vi "Main.vi"() -> ()   [LabVIEW 2019, in "Model.lvlib"]
doc: "This template is based off of the Queued Message Handler design pattern and the Queued Message Handler project template that ships with LabVIEW.\n\nThe main difference is that the queue is private to this module and communication between modules is performed via Broadcast and Request events.\n\nRequest events are wrapped in public API methods and are handled in the Event Handling Loop (EHL) of this VI. Any module can register for Broadcast events sent by this module. The EHL generates messages based on user interface actions.\n\nThe Message Handling Loop (MHL) processes messages generated by the EHL, or by other messages. The messages are string values, so new messages can be added easily to the Message Cases case structure in the MHL. Each message cluster can also provide an optional value for Message Data, which is a variant that can be converted to whatever message-specific data is required.\n_____\nBased on Delacor QMH Project Template 4.2.1.64."
uses:
  Model.lvlib
  <vilib>/Delacor/Delacor QMH/Libraries/Module Admin_class/Delacor_lib_QMH_Module Admin.lvclass
  Module Data--cluster.ctl
  <vilib>/Delacor/Delacor QMH/Libraries/Message Queue_class/Delacor_lib_QMH_Message Queue.lvclass/Delacor_lib_QMH_Message Queue.ctl
  Stop Argument--cluster.ctl
  <vilib>/Delacor/Delacor QMH/Libraries/Module Admin_class/Delacor_lib_QMH_Module Admin.lvclass/Delacor_lib_QMH_Module Admin.ctl
  <vilib>/Delacor/Delacor QMH/Libraries/Message Queue_class/Delacor_lib_QMH_Enqueue Message (Single).vi
  <vilib>/Delacor/Delacor QMH/Libraries/Module Admin_class/Delacor_lib_QMH_Get External Launch.vi
  <vilib>/Utility/error.llb/Error Cluster From Error Code.vi
  <vilib>/ErrorRing/Error Ring.xnode
  <vilib>/Delacor/Delacor QMH/Libraries/Message Queue_class/Delacor_lib_QMH_Message Queue.lvclass
  Stock/Stock.lvlib
  Display/Display.lvlib
  Keypad/Keypad.lvlib
  Money/Money.lvlib
panel:
  in  "Power":bool
  in  "Simulate MHL Error":bool
  in  "Simulate EHL Error":bool
  in  "Module Admin":refnum<class "Delacor_lib_QMH_Module Admin.lvclass">
  out "Status":string
  out "error out":errorcluster
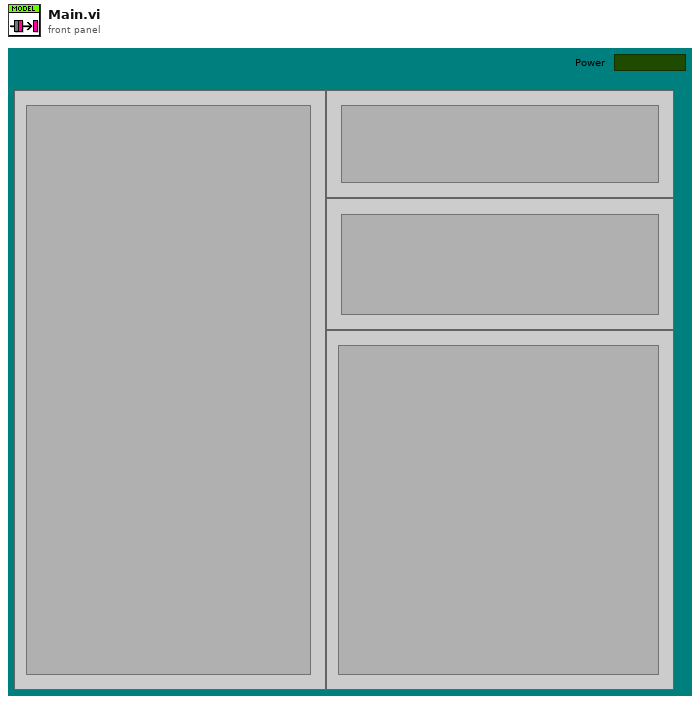
[diagram p1: front panel]
types:
  T1 = typedef "Model.lvlib/Request Events--cluster.ctl" = cluster{"Stop Module":refnum<user-event>, "Show Panel":refnum<user-event>, "Hide Panel":refnum<user-event>, "Get Module Execution Status":refnum<user-event>, "Show Diagram":refnum<user-event>}
  T2 = typedef "Stock.lvlib/Broadcast Events--cluster.ctl" = cluster{"Module Did Init":refnum<user-event>, "Status Updated":refnum<user-event>, "Error Reported":refnum<user-event>, "Module Did Stop":refnum<user-event>, "Update Module Execution Status":refnum<user-event>}
  T3 = typedef "Display.lvlib/Broadcast Events--cluster.ctl" = cluster{"Module Did Init":refnum<user-event>, "Status Updated":refnum<user-event>, "Error Reported":refnum<user-event>, "Module Did Stop":refnum<user-event>, "Update Module Execution Status":refnum<user-event>}
  T4 = typedef "Keypad.lvlib/Broadcast Events--cluster.ctl" = cluster{"Module Did Init":refnum<user-event>, "Status Updated":refnum<user-event>, "Error Reported":refnum<user-event>, "Module Did Stop":refnum<user-event>, "Update Module Execution Status":refnum<user-event>, "Product Selected":refnum<user-event>, "Cancel Request":refnum<user-event>}
  T5 = typedef "Money.lvlib/Broadcast Events--cluster.ctl" = cluster{"Module Did Init":refnum<user-event>, "Status Updated":refnum<user-event>, "Error Reported":refnum<user-event>, "Module Did Stop":refnum<user-event>, "Update Module Execution Status":refnum<user-event>, "Money Entered":refnum<user-event>, "Money Refunded":refnum<user-event>}
  T6 = typedef "Model.lvlib/Module Data--cluster.ctl" = cluster{"Status":string}
  T7 = enum32{"invalid lock state", "Not Locked", "Locked (No Password)", "Password-protected"}
  T8 = typedef "Model.lvlib/Stop Argument--cluster.ctl" = cluster{"Origin":string, "Exit via Stop Module Req?":bool, "Wait for Module to stop?":bool}
  T9 = enum32{"Invalid", "Standard", "Closed", "Hidden", "Minimized", "Maximized"}
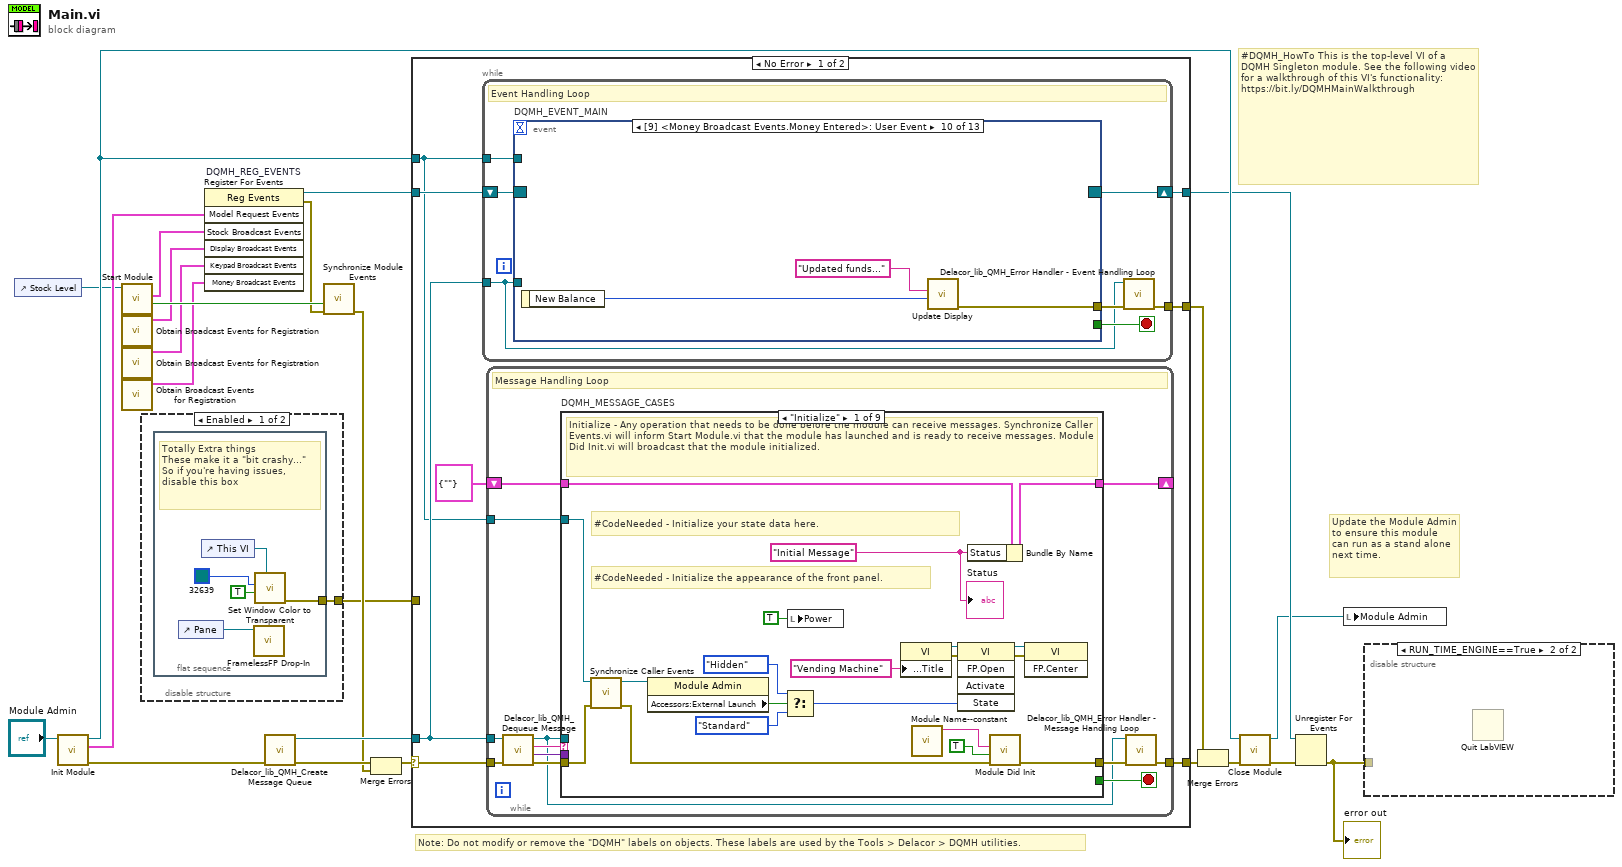
[diagram p0: block diagram]
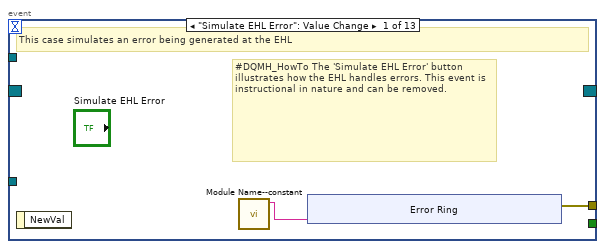
[diagram p4: hidden frame]
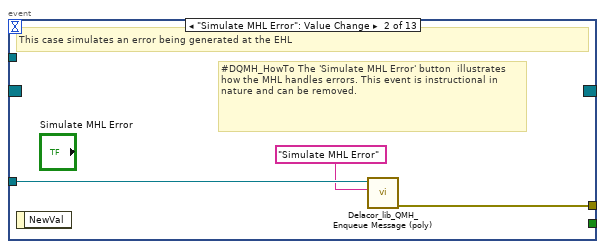
[diagram p5: hidden frame]
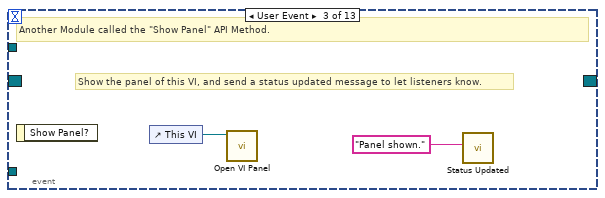
[diagram p6: hidden frame]
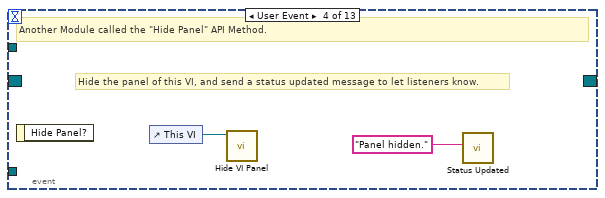
[diagram p7: hidden frame]
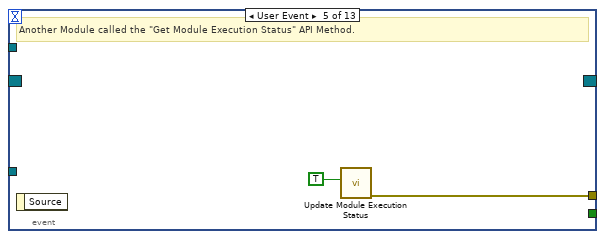
[diagram p8: hidden frame]
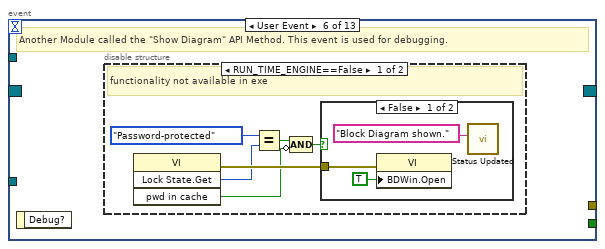
[diagram p9: hidden frame]
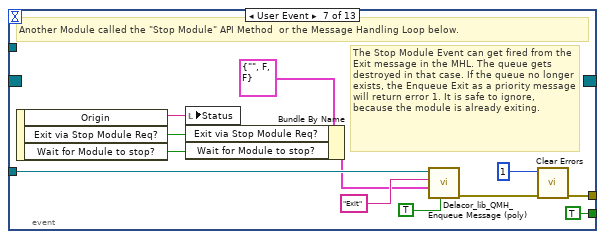
[diagram p12: hidden frame]
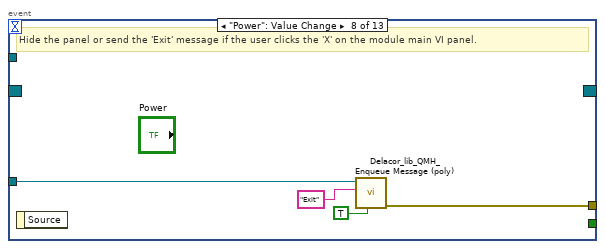
[diagram p13: hidden frame]
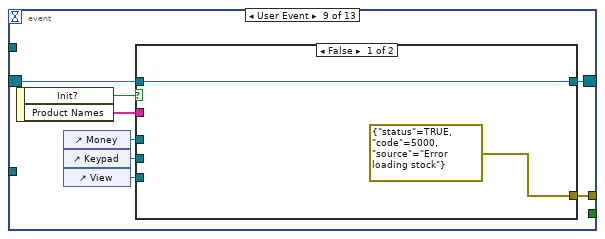
[diagram p14: hidden frame]
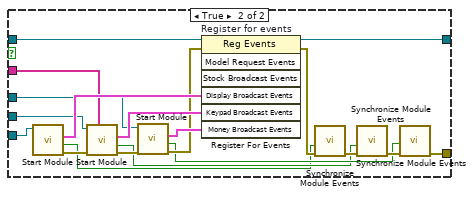
[diagram p15: hidden frame]
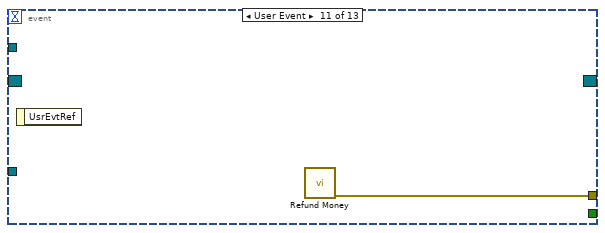
[diagram p16: hidden frame]
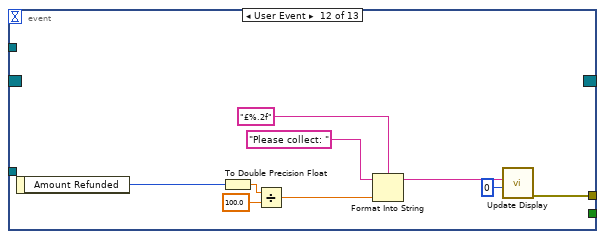
[diagram p17: hidden frame]
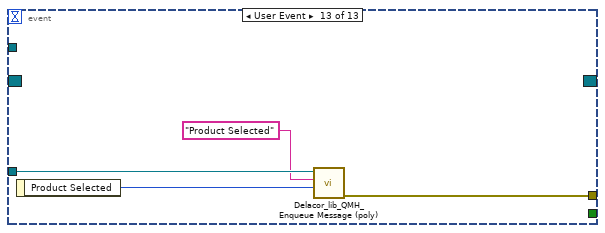
[diagram p18: hidden frame]
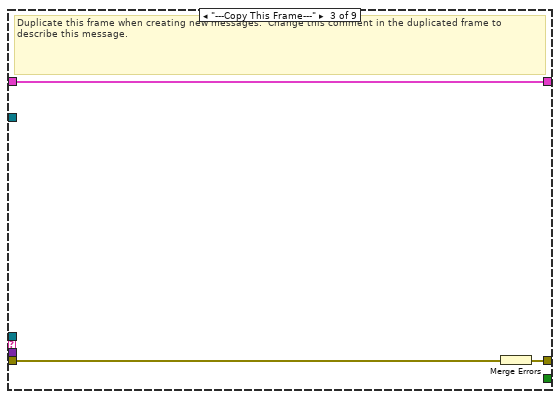
[diagram p20: hidden frame]
diagram:
  # "#DQMH_HowTo This is the top-level VI of a DQMH Singleton module. See the following video for a walkthrough of this VI's functionality: https://bit.ly/DQMHMainWalkthrough"
  # "Note: Do not modify or remove the \"DQMH\" labels on objects. These labels are used by the Tools > Delacor > DQMH utilities."
  # "Update the Module Admin to ensure this module can run as a stand alone next time."
  n1 = control-ref of="Stock Level"() -> (w3:refnum<vi>)
  n2 = call "Init Module.vi"("Singleton Module Admin in"="Module Admin") -> ("error out"=w23:errorcluster, "Model Request Events"=w14:T1, "Singleton Module Admin out"=w17:refnum<class "Delacor_lib_QMH_Module Admin.lvclass">)  [unwired: 8 in]
  n3 = call "Start Module.vi"("Subpanel Ref"=w3) -> ("Wait for Event Sync?"=w9:bool, "Stock Broadcast Events"=w10:T2)  [unwired: 7 in, 2 out]
  n4 = call "Obtain Broadcast Events for Registration.vi"() -> ("Display Broadcast Events"=w6:T3)  [unwired: 9 in, 2 out]
  n5 = call "Obtain Broadcast Events for Registration.vi"() -> ("Keypad Broadcast Events"=w5:T4)  [unwired: 9 in, 2 out]
  n6 = call "Obtain Broadcast Events for Registration.vi"() -> ("Money Broadcast Events"=w4:T5)  [unwired: 9 in, 2 out]
  n7 = disable-structure shown="Enabled" {
    disable-tunnel: [w25 _] -> w1
    frame Enabled {
      n8 = flat-sequence {
        tunnel: [w26] -> w25
        frame #0 {
          # "Totally Extra things\nThese make it a \"bit crashy...\"\nSo if you're having issues, disable this box"
          n9 = control-ref of="Pane"() -> (w30:refnum<vi>)
          n10 = control-ref of="This VI"() -> (w29:refnum<vi>)
          n11 = call "FramelessFP Drop-In.vi"("Pane in"=w30) -> ()  [unwired: 10 in, 1 out]
          n12 = call "Set Window Color to Transparent.vi"("Calling VI's reference"=w29, "Activate"=TRUE, "Color to Replace"=u32 32639) -> ("error out"=w26:errorcluster)  [unwired: 5 in]
        }
      }
    }
    frame Disabled {
    }
  }
  n13 = register-events "DQMH_REG_EVENTS"(w14, w10, w6, w5, w4) -> (reference out=w15:refnum<event-registration>, error out=w8:errorcluster)  [unwired: 2 in]
  n14 = call <vilib>:"Delacor_lib_QMH_Create Message Queue.vi"("error in (no error)"=w23) -> ("error out"=w19:errorcluster, "Message Queue"=w13:refnum<class "Delacor_lib_QMH_Message Queue.lvclass">)  [unwired: 9 in]
  n15 = call "Synchronize Module Events.vi"("error in (no error)"=w8, "Wait for Event Sync?"=w9) -> ("error out"=w7:errorcluster)  [unwired: 9 in]
  n16 = Merge Errors(w19, w7) -> (w18:errorcluster)
  n17 = case shown="No Error" w18 {
    selector: w18 -> [w36 w241]
    tunnel: [w38 w241] -> w24
    tunnel: [w35 w238] -> w16
    tunnel: w15 -> [w33 w238]
    tunnel: w13 -> [w32 _]
    tunnel: [w37 _] -> w21
    tunnel: w17 -> [w31 w234]
    tunnel: w1 -> [_ _]
    frame No Error {
      n18 = while {
        tunnel: w32 -> [w39]
        shift-right: [w42] -> w35
        shift-left: w33 -> [w43]
        tunnel: [w44] -> w37
        tunnel: w31 -> [w40]
        stop <- w41 stop-if-true
        # "Event Handling Loop"
        n19 = event "DQMH_EVENT_MAIN" shown="[9] <Money Broadcast Events.Money Entered>: User Event" {
          selector: w43 -> [_ _ _ _ _ _ _ _ w93 _ _ _ _]
          dyn-events: [_ _ _ _ _ _ _ _ w92 _ _ _ _] -> w42
          timeout: _ -> [_ _ _ _ _ _ _ _ _ _ _ _ _]
          tunnel: [_ _ _ _ _ _ TRUE ("Discard?") _ _ _ _ _ _] -> w41
          tunnel: w39 -> [_ w56 _ _ _ _ w80 w87 _ _ _ _ w134]
          tunnel: [w47 w57 _ _ w63 _ w83 w88 w95 w120 w121 w130 w133] -> w45
          tunnel: w40 -> [_ _ _ _ _ _ _ _ _ _ _ _ _]
          event "Simulate EHL Error": Value Change {
            # "#DQMH_HowTo The 'Simulate EHL Error' button  illustrates how the EHL handles errors. This event is instructional in nature and can be removed."
            # "This case simulates an error being generated at the EHL"
            n20 = event-data() -> ()  [unwired: 1 in, 1 out]
            n21 = call "Module Name--constant.vi"() -> ("Module Name"=w46:string)  [unwired: 11 in]
            n22 = xnode "Error Ring"("parameter 0"=w46) -> ("error out"=w47:errorcluster)
          }
          event "Simulate MHL Error": Value Change {
            # "#DQMH_HowTo The 'Simulate MHL Error' button  illustrates how the MHL handles errors. This event is instructional in nature and can be removed."
            # "This case simulates an error being generated at the EHL"
            n23 = event-data() -> ()  [unwired: 1 in, 1 out]
            n24 = call-poly <vilib>:"Delacor_lib_QMH_Enqueue Message (poly).vi"("Message"="Simulate MHL Error", "Message Queue in"=w56) -> ("error out"=w57:errorcluster)  [unwired: 8 in, 1 out]
          }
          event User Event {
            # "Show the panel of this VI, and send a status updated message to let listeners know."
            # "Another Module called the \"Show Panel\" API Method."
            n25 = event-data() -> ()  [unwired: 1 in, 1 out]
            n26 = control-ref of="This VI"() -> (w59:refnum<vi>)
            n27 = call "Open VI Panel.vi"("VI"=w59) -> ()  [unwired: 10 in, 1 out]
            n28 = call "Status Updated.vi"("Status"="Panel shown." ("format string")) -> ()  [unwired: 10 in, 1 out]
          }
          event User Event {
            # "Hide the panel of this VI, and send a status updated message to let listeners know."
            # "Another Module called the \"Hide Panel\" API Method."
            n29 = event-data() -> ()  [unwired: 1 in, 1 out]
            n30 = control-ref of="This VI"() -> (w61:refnum<vi>)
            n31 = call "Hide VI Panel.vi"("VI"=w61) -> ()  [unwired: 10 in, 1 out]
            n32 = call "Status Updated.vi"("Status"="Panel hidden." ("format string")) -> ()  [unwired: 10 in, 1 out]
          }
          event User Event {
            # "Another Module called the \"Get Module Execution Status\" API Method."
            n33 = event-data() -> ()  [unwired: 1 in, 1 out]
            n34 = call "Update Module Execution Status.vi"("Running?"=TRUE) -> ("error out"=w63:errorcluster)  [unwired: 10 in]
          }
          event User Event {
            # "Another Module called the \"Show Diagram\" API Method. This event is used for debugging."
            n35 = event-data() -> ()  [unwired: 1 in, 1 out]
            n36 = disable-structure shown="RUN_TIME_ENGINE==False" {
              frame condition #0 (active) {
                # "functionality not available in exe"
                n37 = invoke class="VI" method="Lock State.Get"() -> (error out=w69:errorcluster, "Get Lock State"=w68:T7, "pwd in cache"=w65:bool)  [unwired: 4 in, 1 out]
                n38 = Equal?(x=T7."Password-protected", y=w68) -> (x = y?=w66:bool)
                n39 = Compound Arithmetic op=AND(w66, invert w65) -> (w64:bool)
                n40 = case shown="False" w64 {
                  tunnel: w69 -> [w72 _]
                  frame False {
                    n41 = property class="VI"(error in=w72, "BDWin.Open"=TRUE ("Block Diagram Window:Open")) -> ()  [unwired: 1 in, 2 out]
                    n42 = call "Status Updated.vi"("Status"="Block Diagram shown." ("format string")) -> ()  [unwired: 10 in, 1 out]
                  }
                  frame True {
                    # "Password-protected VI, and the password is not in the cache. Do not show the diagram."
                  }
                }
              }
              frame condition #1 {
              }
            }
          }
          event User Event {
            # "The Stop Module Event can get fired from the Exit message in the MHL. The queue gets destroyed in that case. If the queue no longer exists, the Enqueue Exit as a priority message will return error 1. It is safe to ignore, because the module is already exiting."
            # "Another Module called the \"Stop Module\" API Method  or the Message Handling Loop below."
            n43 = event-data() -> ("Origin"=w79:string, "Exit via Stop Module Req?"=w75:bool, "Wait for Module to stop?"=w74:bool)  [unwired: 1 in]
            n44 = local write "Status"(w79) -> ()
            n45 = Bundle By Name(cluster=T8 {"Origin"="", "Exit via Stop Module Req?"=FALSE, "Wait for Module to stop?"=FALSE} ("Stop Argument"), "Exit via Stop Module Req?"=w75, "Wait for Module to stop?"=w74) -> (w73:T8)
            n46 = call-poly <vilib>:"Delacor_lib_QMH_Enqueue Message (poly).vi"("Priority Message? (F)"=TRUE, "Message Data"=w73, "Message"="Exit", "Message Queue in"=w80) -> ("error out"=w84:errorcluster)  [unwired: 6 in, 1 out]
            n47 = call <vilib>:"Clear Errors.vi"("error in (no error)"=w84, "specific error code to clear (0: all)"=1) -> ("error out"=w83:errorcluster)  [unwired: 4 in, 1 out]
          }
          event "Power": Value Change {
            # "Hide the panel or send the 'Exit' message if the user clicks the 'X' on the module main VI panel."
            n48 = event-data() -> ()  [unwired: 1 in, 1 out]
            n49 = call-poly <vilib>:"Delacor_lib_QMH_Enqueue Message (poly).vi"("Priority Message? (F)"=TRUE, "Message"="Exit", "Message Queue in"=w87) -> ("error out"=w88:errorcluster)  [unwired: 7 in, 1 out]
          }
          event User Event {
            n50 = event-data() -> ("Init?"=w96:bool, "Product Names"=w94:string[])  [unwired: 1 in]
            n51 = control-ref of="Money"() -> (w91:refnum<vi>)
            n52 = control-ref of="Keypad"() -> (w90:refnum<vi>)
            n53 = control-ref of="View"() -> (w89:refnum<vi>)
            n54 = case shown="False" w96 {
              tunnel: [errorcluster {"status"=TRUE, "code"=5000, "source"="Error loading stock"} ("error constant") w106] -> w95
              tunnel: w94 -> [_ w102]
              tunnel: w93 -> [w97 w117]
              tunnel: [w97 w116] -> w92
              tunnel: w91 -> [_ w99]
              tunnel: w90 -> [_ w100]
              tunnel: w89 -> [_ w101]
              frame False {
              }
              frame True {
                n55 = call "Start Module.vi"("Subpanel Ref"=w101) -> ("error out"=w112:errorcluster, "Wait for Event Sync?"=w103:bool, "Display Broadcast Events"=w115:T3)  [unwired: 7 in, 1 out]
                n56 = call "Start Module.vi"("Product Names"=w102, "error in (no error)"=w112, "Subpanel Ref"=w100) -> ("error out"=w111:errorcluster, "Wait for Event Sync?"=w104:bool, "Keypad Broadcast Events"=w114:T4)  [unwired: 5 in, 1 out]
                n57 = call "Start Module.vi"("error in (no error)"=w111, "Subpanel Ref"=w99) -> ("error out"=w110:errorcluster, "Wait for Event Sync?"=w105:bool, "Money Broadcast Events"=w113:T5)  [unwired: 6 in, 1 out]
                n58 = register-events "Register for events"(reference=w117, error in=w110, w115, w114, w113) -> (reference out=w116:refnum<event-registration>, error out=w109:errorcluster)  [unwired: 2 in]
                n59 = call "Synchronize Module Events.vi"("error in (no error)"=w109, "Wait for Event Sync?"=w103) -> ("error out"=w108:errorcluster)  [unwired: 9 in]
                n60 = call "Synchronize Module Events.vi"("error in (no error)"=w108, "Wait for Event Sync?"=w104) -> ("error out"=w107:errorcluster)  [unwired: 9 in]
                n61 = call "Synchronize Module Events.vi"("error in (no error)"=w107, "Wait for Event Sync?"=w105) -> ("error out"=w106:errorcluster)  [unwired: 9 in]
              }
            }
          }
          event User Event {
            n62 = event-data() -> ("New Balance"=w119:u32)  [unwired: 1 in]
            n63 = call "Update Display.vi"("Balance"=w119, "Message to display"="Updated funds...") -> ("error out"=w120:errorcluster)  [unwired: 9 in]
          }
          event User Event {
            n64 = event-data() -> ()  [unwired: 1 in, 1 out]
            n65 = call "Refund Money.vi"() -> ("error out"=w121:errorcluster)  [unwired: 11 in]
          }
          event User Event {
            n66 = event-data() -> ("Amount Refunded"=w124:u32)  [unwired: 1 in]
            n67 = To Double Precision Float(number=w124) -> (double precision float=w127:dbl)
            n68 = Divide(x=w127, y=100.0) -> (x/y=w125:dbl)
            n69 = Format Into String(format string="£%.2f", initial string="Please collect: ", w125) -> (resulting string=w123:string)  [unwired: 1 in, 1 out]
            n70 = call "Update Display.vi"("Balance"=u32 0, "Message to display"=w123) -> ("error out"=w130:errorcluster)  [unwired: 9 in]
          }
          event User Event {
            n71 = event-data() -> ("Product Selected"=w131:u32)  [unwired: 1 in]
            n72 = call-poly <vilib>:"Delacor_lib_QMH_Enqueue Message (poly).vi"("Message Data"=w131, "Message"="Product Selected", "Message Queue in"=w134) -> ("error out"=w133:errorcluster)  [unwired: 7 in, 1 out]
          }
        }
        n73 = call-dynamic "Delacor_lib_QMH_Error Handler - Event Handling Loop.vi"("error in (no error)"=w45, "Message Queue in"=w39) -> ("dup error in"=w44:errorcluster)  [unwired: 8 in, 1 out]
      }
      n74 = while {
        tunnel: w32 -> [w137]
        shift-right: [w141] -> _
        shift-left: T6 {"Status"=""} ("Data Cluster") -> [w142]
        tunnel: w36 -> [w145]
        tunnel: [w143] -> w38
        tunnel: w31 -> [w135]
        stop <- w140 stop-if-true
        # "Message Handling Loop"
        n75 = call-dynamic "Delacor_lib_QMH_Dequeue Message.vi"("error in (no error)"=w145, "Message Queue in"=w137) -> ("error out"=w144:errorcluster, "Message Data"=w138:variant, "Message"=w139:string, "Message Queue out"=w136:refnum<class "Delacor_lib_QMH_Message Queue.lvclass">)  [unwired: 6 in]
        n76 = case "DQMH_MESSAGE_CASES" shown="\"Initialize\"" w139 {
          selector: w139 -> [_ _ _ _ _ _ _ _ w221]
          tunnel: w136 -> [_ _ _ _ _ _ w196 w213 _]
          tunnel: w144 -> [w164 w168 w171 w176 w180 w185 w203 w219 w223]
          tunnel: [w162 w168 w170 w172 w180 w184 w199 w216 w224] -> w146
          tunnel: w142 -> [w154 w167 w169 w178 w179 w182 w198 w212 w222]
          tunnel: [w153 w167 w169 w178 w179 w182 w198 w212 w222] -> w141
          tunnel: [_ _ _ _ _ _ _ w211 _] -> w140
          tunnel: w138 -> [_ _ _ w177 _ _ w197 w210 _]
          tunnel: w135 -> [w155 _ _ _ _ _ w195 w205 _]
          frame "Initialize" {
            w149 = "Initial Message" ("Initial Message")
            # "#CodeNeeded - Initialize the appearance of the front panel."
            # "#CodeNeeded - Initialize your state data here."
            # "Initialize - Any operation that needs to be done before the module can receive messages. Synchronize Caller Events.vi will inform Start Module.vi that the module has launched and is ready to receive messages. Module Did Init.vi will broadcast that the module initialized."
            n77 = call "Synchronize Caller Events.vi"("error in (no error)"=w164, "Singleton Module Admin in"=w155) -> ("error out"=w163:errorcluster, "Singleton Module Admin out"=w150:refnum<class "Delacor_lib_QMH_Module Admin.lvclass">)  [unwired: 8 in]
            n78 = property class="Module Admin"(reference=w150) -> ("Accessors:External Launch"=w159:bool)  [unwired: 1 in, 2 out]
            n79 = Select(t=T9."Hidden" ("State"), s=w159, f=T9."Standard" ("State")) -> (s? t:f=w156:T9)
            n80 = local write "Power"(TRUE ("Power")) -> ()
            n81 = property class="VI"("Front Panel.Title"="Vending Machine" ("Front Panel Window:Title")) -> (reference out=w161:refnum<vi>, error out=w166:errorcluster)  [unwired: 2 in]
            n82 = call "Module Name--constant.vi"() -> ("Module Name"=w151:string)  [unwired: 11 in]
            n83 = invoke class="VI" method="FP.Open"(reference=w161, error in=w166, "State"=w156) -> (reference out=w160:refnum<vi>, error out=w165:errorcluster)  [unwired: 2 in, 3 out]
            n84 = Bundle By Name(cluster=w154, "Status"=w149) -> (w153:T6)
            n85 = call "Module Did Init.vi"("error in (no error)"=w163, "Initialized?"=TRUE, "Origin"=w151) -> ("error out"=w162:errorcluster)  [unwired: 8 in]
            n86 = invoke class="VI" method="FP.Center"(reference=w160, error in=w165) -> ()  [unwired: 1 in, 3 out]
            "Status" <- w149
          }
          frame "--- Module Specific ---" {
            # "Separator -- The following cases handle messages specific to this Module."
          }
          frame "---Copy This Frame---" {
            # "Duplicate this frame when creating new messages.  Change this comment in the duplicated frame to describe this message."
            n87 = Merge Errors(w171) -> (w170:errorcluster)
          }
          frame "Product Selected" {
            # "All in one VI to reduce the risk of race conditions"
            # "Check Stock Level, Check Balance\nOutputs: Not in stock,  Insufficient Funds, Accepted (Reduce Stock and Balance"
            n88 = Variant To Data(error in=w176, type=u32 0 ("Product Selected"), Variant=w177) -> (data=w174:u32, error out=w173:errorcluster)
            n89 = call "Despence Product.vi"("error in (no error)"=w173, "Stock Item"=w174) -> ("error out"=w172:errorcluster)  [unwired: 9 in]
          }
          frame "--- Exit and Error Handling---" {
            # "Separator - The following cases handle errors and exit messages."
          }
          frame "Simulate MHL Error" {
            # "#DQMH_HowTo The 'Simulate MHL Error' button  illustrates how the MHL handles errors. This event is instructional in nature and can be removed."
            # "Simulate an error occurring at the MHL"
            n90 = call "Module Name--constant.vi"() -> ("Module Name"=w181:string)  [unwired: 11 in]
            n91 = xnode "Error Ring"("parameter 0"=w181) -> ("error out"=w183:errorcluster)
            n92 = Merge Errors(w185, w183) -> (w184:errorcluster)
          }
          frame "Error" {
            # "If the module is running standalone, then pop up an error dialog and call the \"Exit\" message."
            # "#CodeRecommended - If you ever change the name of this \"Error\" message, you'll need to update the name in the Check Loop Error.vi as well."
            # "#CodeRecommended - If the module is running in standalone mode (External Launch = FALSE), this code will pop up an error dialog and call the 'Exit' message if an error occurs. Add more fine-grained error handling here."
            # "Error - Check the error message data and respond accordingly. This message is sent by the \"Error Handler\" VIs at the end of each loop in this application."
            n93 = property class="Module Admin" props=["Accessors:External Launch"](reference=w195) -> ()  [unwired: 1 in, 3 out]
            n94 = Variant To Data(error in=w203, type=errorcluster {"status"=FALSE, "code"=0, "source"=""} ("error constant"), Variant=w197) -> (data=w204:errorcluster, error out=w201:errorcluster)
            n95 = call "Error Reported.vi"("Error"=w204) -> ()  [unwired: 10 in, 1 out]
            n96 = call <vilib>:"Simple Error Handler.vi"("error in (no error)"=w204) -> ()  [unwired: 4 in, 5 out]
            n97 = call-poly <vilib>:"Delacor_lib_QMH_Enqueue Message (poly).vi"("Priority Message? (F)"=TRUE, "Message"="Exit", "Message Queue in"=w196) -> ("error out"=w200:errorcluster)  [unwired: 7 in, 1 out]
            n98 = Merge Errors(w201, w200) -> (w199:errorcluster)
            n99 = local write "error out"(w199) -> ()
          }
          frame "Exit" {
            w209 = 91  # 91: not all Exit messages will have an argument
            w211 = TRUE  # Stop the VI
            # "Release the message queue reference"
            # "Exit - Exit the application."
            n100 = Variant To Data(error in=w219, type=T8 {"Origin"="", "Exit via Stop Module Req?"=FALSE, "Wait for Module to stop?"=FALSE} ("Stop Argument"), Variant=w210) -> (data=w207:T8, error out=w215:errorcluster)
            n101 = call <vilib>:"Clear Errors.vi"("error in (no error)"=w215, "specific error code to clear (0: all)"=w209) -> ("error out"=w218:errorcluster)  [unwired: 4 in, 1 out]
            n102 = control-ref of="This VI"() -> (w206:refnum<vi>)
            n103 = call-dynamic "Delacor_lib_QMH_Release Message Queue.vi"("error in (no error)"=w218, "Message Queue"=w213) -> ("error out"=w217:errorcluster)  [unwired: 9 in]
            n104 = call "Handle Exit.vi"("Stop Argument"=w207, "Admin in"=w205, "VI reference"=w206) -> ("error out"=w214:errorcluster)  [unwired: 7 in, 1 out]
            n105 = Merge Errors(w217, w214) -> (w216:errorcluster)
            n106 = call "Stop Module.vi"() -> ()  [unwired: 11 in, 1 out]
            n107 = call "Stop Module.vi"() -> ()  [unwired: 11 in, 1 out]
            n108 = call "Stop Module.vi"() -> ()  [unwired: 11 in, 1 out]
            n109 = call "Stop Module.vi"() -> ()  [unwired: 11 in, 1 out]
          }
          frame Default {
            # "'Default' case only runs if there is a message that isn't defined in any of the other cases.  Output a programming error."
            n110 = call "Module Name--constant.vi"() -> ("Module Name"=w220:string)  [unwired: 11 in]
            n111 = xnode "Error Ring"("parameter 0"=w221, "parameter 1"=w220) -> ("error out"=w225:errorcluster)
            n112 = Merge Errors(w223, w225) -> (w224:errorcluster)
          }
        }
        n113 = call-dynamic "Delacor_lib_QMH_Error Handler - Message Handling Loop.vi"("error in (no error)"=w146, "Message Queue in"=w136) -> ("dup error in"=w143:errorcluster)  [unwired: 8 in, 1 out]
      }
    }
    frame Error {
      # "Synchronize Caller Events.vi will inform Start Module.vi that the module has launched and will let the code calling Start Module.vi register for broadcasts and would permit the caller receive the broadcast that an error occurred at launch time."
      n114 = call "Synchronize Caller Events.vi"("Singleton Module Admin in"=w234) -> ("error out"=w239:errorcluster)  [unwired: 9 in, 1 out]
      n115 = call "Module Name--constant.vi"() -> ("Module Name"=w237:string)  [unwired: 11 in]
      n116 = Format Into String(format string="An error occurred during initialization. %s is no longer running.", w237) -> (resulting string=w235:string)  [unwired: 2 in, 1 out]
      n117 = Merge Errors(w241, w239) -> (w240:errorcluster)
      n118 = call "Error Reported.vi"("Additional Information"=w235, "Error"=w240) -> ()  [unwired: 9 in, 1 out]
    }
  }
  n119 = Merge Errors(w21, w24) -> (w20:errorcluster)
  n120 = call "Close Module.vi"("error in (no error)"=w20, "Module Admin in"=w17) -> ("error out"=w22:errorcluster, "Module Admin out"=w11:refnum<class "Delacor_lib_QMH_Module Admin.lvclass">)  [unwired: 7 in, 1 out]
  n121 = Unregister For Events(event registration refnum=w16, error in=w22) -> (error out=w2:errorcluster)
  "error out" <- w2
  n122 = local write "Module Admin"(w11) -> ()
  n123 = disable-structure shown="RUN_TIME_ENGINE==True" {
    disable-tunnel: w2 -> [_ _]
    frame condition #0 (active) {
    }
    frame condition #1 {
      n124 = Quit LabVIEW() -> ()  [unwired: 1 in]
    }
  }
